vi "Experiment 22.vi"() -> ()   [LabVIEW 2026]
doc: "This VI (Experiment 22) was created as a Save As... copy of Experiment 4."
uses:
  <vilib>/Analysis/baseanly.llb/Mean (DBL).vi
  <vilib>/Analysis/NI_AALBase.lvlib
panel:
  out "Execution Time - Per Call (us)":dbl format="%.6f"
  out "Execution Time - 1M Calls (seconds)":dbl format="%.6f"
  out "Output":dbl[](array[numeric]) format="%.3f"
  # "Experiment 22"
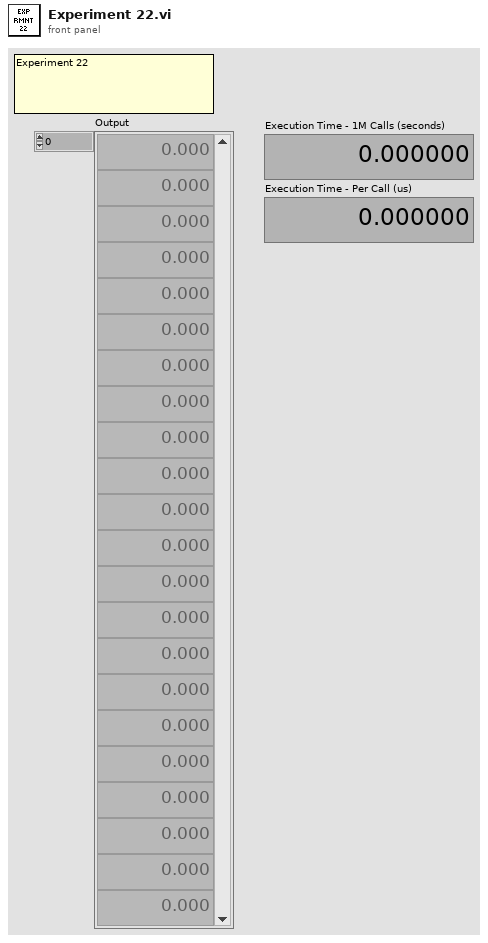
[diagram p1: front panel]
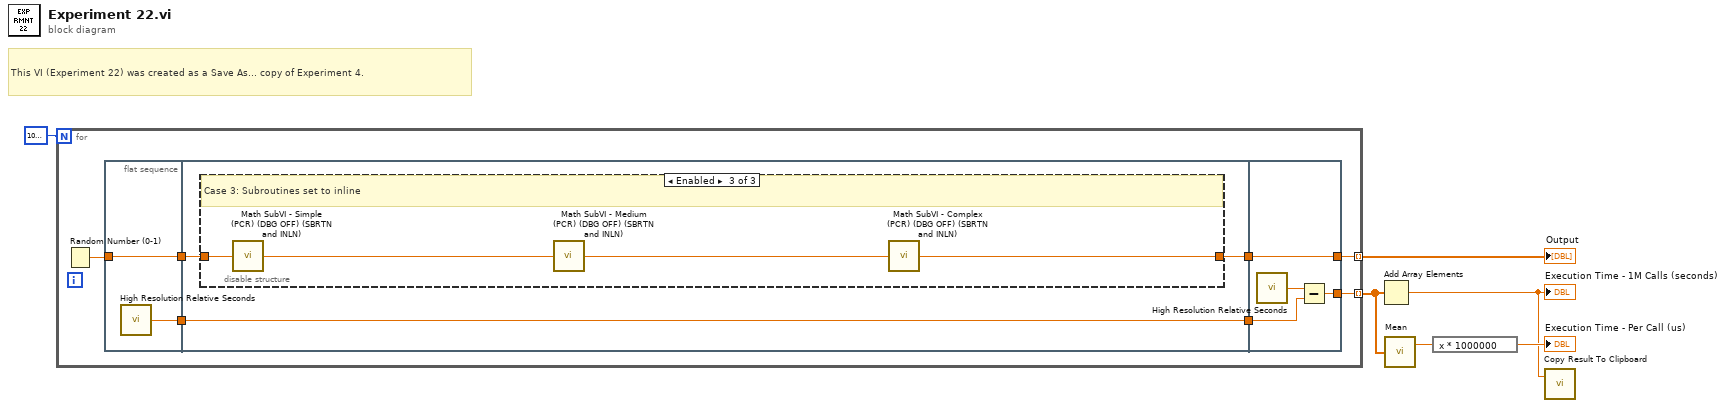
[diagram p0: block diagram]
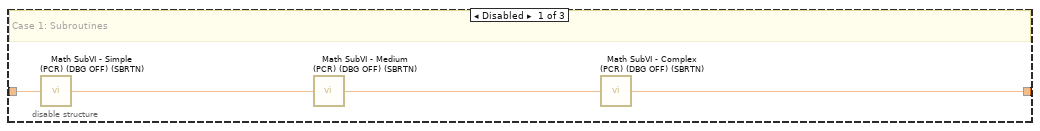
[diagram p2: hidden frame]
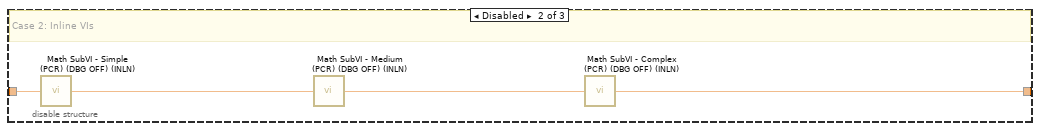
[diagram p3: hidden frame]
diagram:
  # "This VI (Experiment 22) was created as a Save As... copy of Experiment 4."
  n1 = for {
    N: 1000000 -> [_]
    tunnel: [w13] -> w6 mode=indexing
    tunnel: [w7] -> w4 mode=indexing
    n2 = Random Number (0-1)() -> (number: 0 to 1=w12:dbl)
    n3 = flat-sequence {
      tunnel: w12 -> [w15]
      tunnel: [w15] -> w11
      tunnel: [w14] -> w8
      tunnel: w11 -> [w16]
      tunnel: [w17] -> w10
      tunnel: [w18] -> w9
      tunnel: w8 -> [w18]
      tunnel: [w34] -> w13
      tunnel: w10 -> [w34]
      tunnel: w9 -> [w32]
      tunnel: [w31] -> w7
      frame #0 {
        n4 = call <vilib>:"High Resolution Relative Seconds.vi"() -> ("relative seconds"=w14:dbl)
      }
      frame #1 {
        n5 = disable-structure shown="Enabled" {
          disable-tunnel: [w19 w23 w27] -> w17
          disable-tunnel: w16 -> [w21 w25 w29]
          frame Disabled {
            # "Case 1: Subroutines"
            n6 = call "Math SubVI - Simple (PCR) (DBG OFF) (SBRTN).vi"("Input"=w21) -> ("Output"=w22:dbl)
            n7 = call "Math SubVI - Medium (PCR) (DBG OFF) (SBRTN).vi"("Input"=w22) -> ("Output"=w20:dbl)
            n8 = call "Math SubVI - Complex (PCR) (DBG OFF) (SBRTN).vi"("Input"=w20) -> ("Output"=w19:dbl)
          }
          frame Disabled {
            # "Case 2: Inline VIs"
            n9 = call "Math SubVI - Simple (PCR) (DBG OFF) (INLN).vi"("Input"=w25) -> ("Output"=w26:dbl)
            n10 = call "Math SubVI - Medium (PCR) (DBG OFF) (INLN).vi"("Input"=w26) -> ("Output"=w24:dbl)
            n11 = call "Math SubVI - Complex (PCR) (DBG OFF) (INLN).vi"("Input"=w24) -> ("Output"=w23:dbl)
          }
          frame Enabled {
            # "Case 3: Subroutines set to inline"
            n12 = call "Math SubVI - Simple (PCR) (DBG OFF) (SBRTN and INLN).vi"("Input"=w29) -> ("Output"=w30:dbl)
            n13 = call "Math SubVI - Medium (PCR) (DBG OFF) (SBRTN and INLN).vi"("Input"=w30) -> ("Output"=w28:dbl)
            n14 = call "Math SubVI - Complex (PCR) (DBG OFF) (SBRTN and INLN).vi"("Input"=w28) -> ("Output"=w27:dbl)
          }
        }
      }
      frame #2 {
        n15 = call <vilib>:"High Resolution Relative Seconds.vi"() -> ("relative seconds"=w33:dbl)
        n16 = Subtract(x=w33, y=w32) -> (x-y=w31:dbl)
      }
    }
  }
  "Output" <- w6
  n17 = Add Array Elements(numeric array=w4) -> (sum=w1:dbl)
  "Execution Time - 1M Calls (seconds)" <- w1
  n18 = call-poly <vilib>:"Mean.vi"("X"=w4) -> ("mean"=w3:dbl)  [unwired: 1 out]
  n19 = expression code="x * 1000000"(w3) -> (→"Execution Time - Per Call (us)":dbl)
  n20 = call "Copy Result To Clipboard.vi"("Input"=w1) -> ()  [unwired: 1 in]
